vi "mean.vi"(11 "parameters":dbl[][](array[numeric])) -> (2 "k":dbl, 3 "b":dbl)   [LabVIEW 2019]
uses:
  <vilib>/Analysis/baseanly.llb/Mean (DBL).vi
  <vilib>/Analysis/NI_AALBase.lvlib
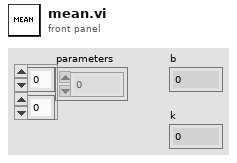
[diagram p1: front panel]
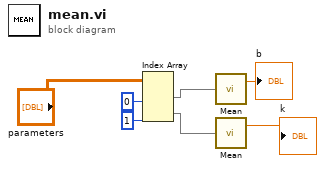
[diagram p0: block diagram]
diagram:
  n1 = Index Array(array="parameters", index (col) #1=0 ("disabled index (col)"), index (col) #2=1 ("index (col)")) -> (element #1=w4:dbl[], element #2=w5:dbl[])  [unwired: 2 in]
  n2 = call-poly <vilib>:"Mean.vi"("X"=w4) -> ("mean"=→"b":dbl)  [unwired: 1 out]
  n3 = call-poly <vilib>:"Mean.vi"("X"=w5) -> ("mean"=→"k":dbl)  [unwired: 1 out]
